vi "Plotter TCP Reader2.vi"(8 "error in":errorcluster, 9 "timeout ms":i32=1000, 10 "TCP index":i32, 11 "references":T1) -> (0 "error out":errorcluster)   [LabVIEW 2013]
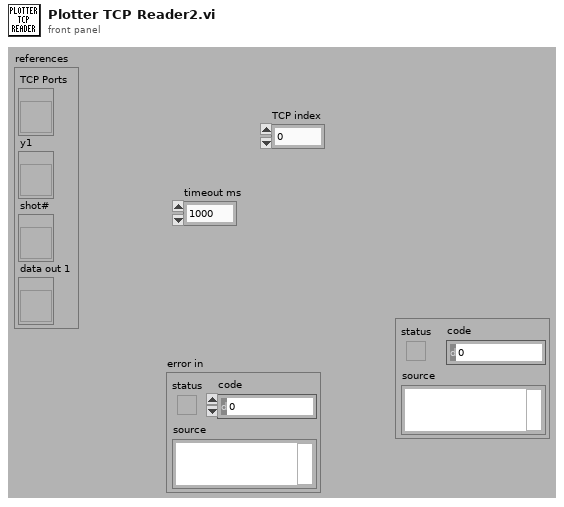
[diagram p1: front panel]
types:
  T1 = cluster{"TCP Ports":refnum<vi>, "y1":refnum<vi>, "shot#":refnum<vi>, "data out 1":refnum<vi>}
  T2 = typedef "Plotter FGV cluster control.ctl" = cluster{"Multicast Address":string, "Plotter Busy":bool, "Plotter Exit":bool, "Mcast Port":u16}
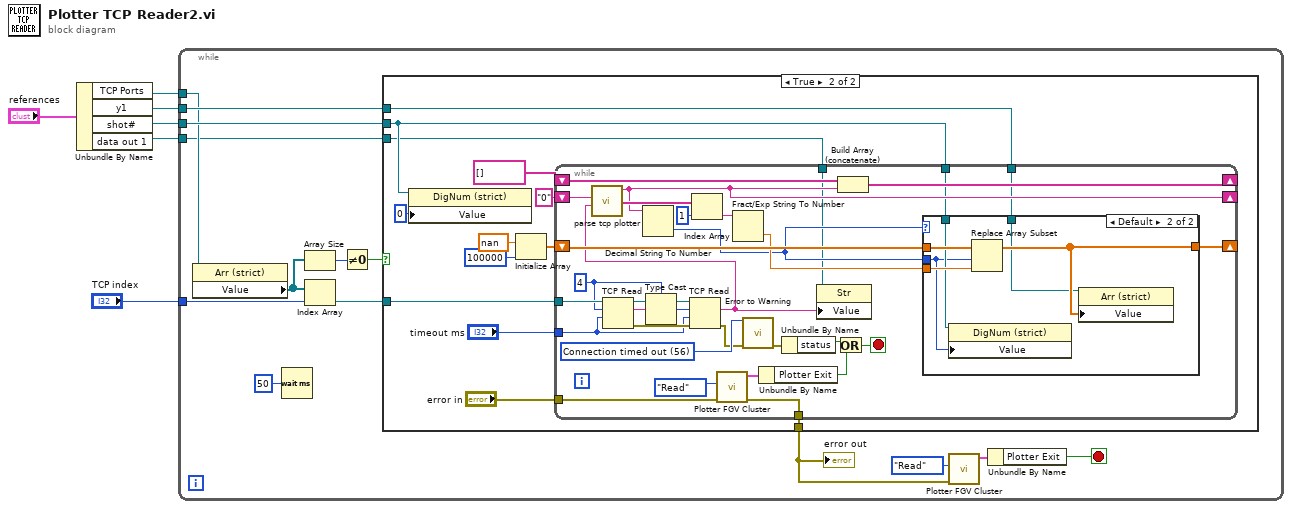
[diagram p0: block diagram]
diagram:
  n1 = Unbundle By Name("references") -> ("TCP Ports"=w4:refnum<vi>, "y1"=w3:refnum<vi>, "shot#"=w2:refnum<vi>, "data out 1"=w1:refnum<vi>)
  n2 = while {
    tunnel: w2 -> [w20]
    tunnel: w3 -> [w19]
    tunnel: w4 -> [w13]
    tunnel: "TCP index" -> [w8]
    tunnel: w1 -> [w7]
    stop <- w15 stop-if-true
    n3 = property class="Arr (strict)"(reference=w13) -> ("Value"=w11:refnum<k5>[])  [unwired: 1 in, 2 out]
    n4 = Wait (ms)(milliseconds to wait=u32 50) -> ()  [unwired: 1 out]
    n5 = Array Size(array=w11) -> (size(s)=w10:i32)
    n6 = Index Array(array=w11, index=w8) -> (element=w12:refnum<k5>)
    n7 = Not Equal To 0?(x=w10) -> (x != 0?=w9:bool)
    n8 = case shown="True" w9 {
      tunnel: w20 -> [_ w25]
      tunnel: w19 -> [_ w24]
      tunnel: [_ w23] -> w16
      tunnel: w12 -> [_ w22]
      tunnel: w7 -> [_ w21]
      frame False {
      }
      frame True {
        n9 = property class="DigNum (strict)"(reference=w25, "Value"=0 ("shot#")) -> ()  [unwired: 1 in, 2 out]
        n10 = Initialize Array(nan ("element"), 100000 ("dimension size")) -> (w27:dbl[])
        n11 = while {
          tunnel: w22 -> [w64]
          tunnel: "timeout ms" -> [w62]
          shift-right: [w46] -> _
          shift-left: "0" ("shot #") -> [w57]
          tunnel: "error in" -> [w53]
          tunnel: [w52] -> w23
          shift-right: [w44] -> _
          shift-left: string[] [] -> [w45]
          shift-right: [w40] -> _
          shift-left: w27 -> [w42]
          tunnel: w25 -> [w38]
          tunnel: w24 -> [w37]
          tunnel: w21 -> [w34]
          stop <- w59 stop-if-true
          w49 = 56 items=["No Error", "Argument Error", "Memory Full", "Out of Zone", "End of File", "File Already Open", "Generic File IO Error", "File Not Found", "File Permission Error", "Disk Full", "Duplicate Path", "Too Many Files Open", "Not Enabled", "Resource File Not Found", "Cannot Add Resource", "Resource Not Found", "Image Not Found", "Image Memory Error", "Pen Does Not Exist", "Config Bad Type", "Config Token Not Found", "Config Parse Error", "Config Memory Error", "Bad External Code Format", "Bad External Code Offset", "External Code Not Present", "Null Window", "Destroy Window Mixup", "Null Menu", "Print Aborted", "Bad Print Record", "Print Driver Error", "Windows Error During Print", "Memory Error During Print", "Print Dialog Error", "Generic Print Error", "Invalid Device Refnum", "Device Not Found", "Device Parameter Error", "Device Unit Error", "Can't Open Device", "Device Call Aborted", "Generic Error", "Cancelled By User", "Object ID Too Low", "Object ID Too High", "Object Not In Heap", "Unknown Heap", "Bad DefProc ID", "DefProc Not In Table", "Message Out Of Range", "Null Method", "Unknown Message", "Manager Call Not Supported", "Bad address", "Connection In progress", "Connection timed out", "Connection is already in progress", "Network attribute not supported", "Network error", "Address in use", "System out of memory", "Connection aborted", "Connection refused", "Connection is not connected", "Connection is already connected", "Connection closed", "Initialize error (interapplication manager)", "Bad occurrence", "Wait on unbound occurrence handler", "Occurrence queue overflow", "Bad path", "Semaphore not signaled", "Unrecognized type (interapplication manager)"] ("1st Error to Convert")
          w36 = 4 ("bytes to read")
          n12 = TCP Read(connection ID=w64, bytes to read=w36, 9:w62) -> (connection ID out=w65:refnum<k5>, data out=w61:string, error out=w63:errorcluster)  [unwired: 2 in]
          n13 = Type Cast(type=w36, x=w61) -> (*(type *) &x=w60:i32)
          n14 = TCP Read(connection ID=w65, bytes to read=w60, error in (no error)=w63, 9:w62) -> (data out=w35:string, error out=w48:errorcluster)  [unwired: 1 in, 1 out]
          n15 = call "parse tcp plotter.vi"("data in"=w35, "shot #"=w57) -> ("variable values"=w51:string[], "shot # out"=w46:string)  [unwired: 8 in]
          n16 = Decimal String To Number(string=w46) -> (number=w39:i32)  [unwired: 2 in, 1 out]
          n17 = Index Array(array=w51, index=1) -> (element=w50:string)
          n18 = call "Plotter FGV Cluster.vi"("error in"=w53, "Function"=enum16{"Read", "Write", "Clear"}."Read") -> ("error out"=w52:errorcluster, "Cluster out"=w55:T2)  [unwired: 8 in]
          n19 = Fract/Exp String To Number(string=w50) -> (number=w41:dbl)  [unwired: 3 in, 1 out]
          n20 = call <vilib>:"Error to Warning.vi"("1st Error to Convert"=w49, "error in"=w48) -> ("warning out"=w47:errorcluster)  [unwired: 13 in]
          n21 = Unbundle By Name(w55) -> ("Plotter Exit"=w54:bool)
          n22 = Unbundle By Name(w47) -> ("status"=w58:bool)
          n23 = property class="Str"(reference=w34, "Value"=w35) -> ()  [unwired: 1 in, 2 out]
          n24 = Or(x=w58, y=w54) -> (x .or. y?=w59:bool)
          n25 = Build Array (concatenate)(w45, w46) -> (w44:string[])
          n26 = case shown="Default" w39 {
            tunnel: w42 -> [w66 w72]
            tunnel: w39 -> [_ w69]
            tunnel: w41 -> [_ w71]
            tunnel: [w66 w68] -> w40
            tunnel: w38 -> [_ w70]
            tunnel: w37 -> [_ w67]
            frame 0 {
            }
            frame Default {
              n27 = property class="DigNum (strict)"(reference=w70, "Value"=w69) -> ()  [unwired: 1 in, 2 out]
              n28 = Replace Array Subset(array=w72, new element=w71, index=w69) -> (w68:dbl[])
              n29 = property class="Arr (strict)"(reference=w67, "Value"=w68) -> ()  [unwired: 1 in, 2 out]
            }
          }
        }
      }
    }
    "error out" <- w16
    n30 = call "Plotter FGV Cluster.vi"("error in"=w16, "Function"=enum16{"Read", "Write", "Clear"}."Read") -> ("Cluster out"=w18:T2)  [unwired: 8 in, 1 out]
    n31 = Unbundle By Name(w18) -> ("Plotter Exit"=w15:bool)
  }
